vi "Przenies aktywne FVG.vi"(7 "Akcja (Get)":T1, 8 "error in (no error)":errorcluster, 10 "DI Aktywne in":bool[](array[boolean])=[TRUE, TRUE, FALSE, TRUE, FALSE, FALSE, FALSE, FALSE], 11 "AI Aktywne in":bool[](array[boolean])=[TRUE, TRUE, FALSE, TRUE, FALSE, FALSE, FALSE, FALSE]) -> (0 "error out":errorcluster, 2 "DI Aktywne out":bool[](array[boolean])=[TRUE, TRUE, FALSE, TRUE, FALSE, FALSE, FALSE, FALSE], 3 "AI Aktywne out":bool[](array[boolean])=[TRUE, TRUE, FALSE, TRUE, FALSE, FALSE, FALSE, FALSE])   [LabVIEW 2013]
doc: "Zmienna funkcjonalna zapamiêtuje i przenosi\nustawienia aktywnoœci kana³ów analogowych i cyfrowych"
uses:
  Kontrolki/FVGs/FVG GUI akcje.ctl
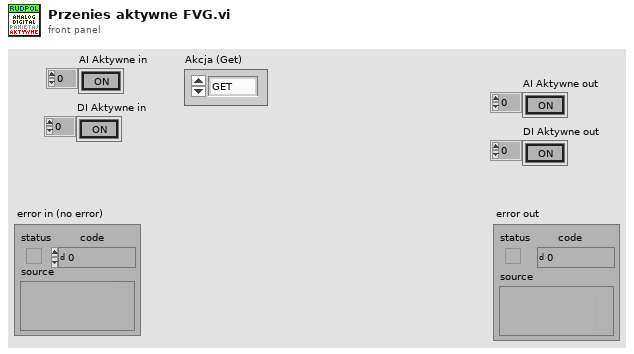
[diagram p1: front panel]
types:
  T1 = typedef "FVG GUI akcje.ctl" = enum16{"GET", "SET AI Aktywny", "SET DI Aktywny"}
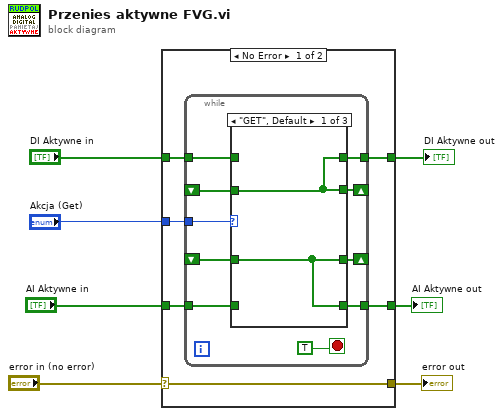
[diagram p0: block diagram]
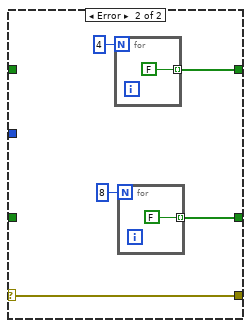
[diagram p4: hidden frame]
diagram:
  n1 = case shown="No Error" "error in (no error)" {
    selector: "error in (no error)" -> [w13 w34]
    tunnel: [w13 w34] -> w6
    tunnel: "Akcja (Get)" -> [w12 _]
    tunnel: "AI Aktywne in" -> [w11 _]
    tunnel: [w10 w32] -> w4
    tunnel: "DI Aktywne in" -> [w9 _]
    tunnel: [w8 w30] -> w1
    frame No Error {
      n2 = while {
        tunnel: w12 -> [w22]
        tunnel: w11 -> [w21]
        shift-right: [w20] -> _
        shift-left: _ -> [w19]
        tunnel: [w18] -> w10
        tunnel: w9 -> [w17]
        shift-right: [w16] -> _
        shift-left: _ -> [w14]
        tunnel: [w15] -> w8
        stop <- TRUE stop-if-true
        n3 = case shown="\"GET\", Default" w22 {
          tunnel: w21 -> [_ w27 _]
          tunnel: [w25 w27 w29] -> w20
          tunnel: w19 -> [w25 _ w29]
          tunnel: [w25 w27 w29] -> w18
          tunnel: w17 -> [_ _ w28]
          tunnel: [w24 w26 w28] -> w16
          tunnel: [w24 w26 w28] -> w15
          tunnel: w14 -> [w24 w26 _]
          frame "GET", Default {
          }
          frame "SET AI Aktywny" {
          }
          frame "SET DI Aktywny" {
          }
        }
      }
    }
    frame Error {
      n4 = for {
        N: 4 -> [_]
        tunnel: [FALSE] -> w30 mode=indexing
      }
      n5 = for {
        N: 8 -> [_]
        tunnel: [FALSE] -> w32 mode=indexing
      }
    }
  }
  "error out" <- w6
  "AI Aktywne out" <- w4
  "DI Aktywne out" <- w1
